vi "PH_Cam_BaseClass.set i Attr and open Services.vi"(0 "i ref in":refnum<vi>, 5 "error in (no error)":errorcluster) -> (14 "i ref out":refnum<vi>, 15 "Image Type":T1 {"Image Type" items=["Grayscale (U8)", "Grayscale (I16)", "Grayscale (SGL)", "Complex (CSG)", "RGB (U32)", "HSL (U32)", "RGB (U64)", "Grayscale (U16)"]}, 16 "i Attributes":T3={"Gui Refs"={"Frame Rate"=refnum, "Get Frame Rate"=refnum, "Show Image"=refnum, "Get Histogram"=refnum, "Mapping"=refnum, "Histogram"=refnum, "Center Cross"=refnum, "Center of Gravity"=refnum, "Scale Factor [%]"=refnum, "Save Image"=refnum, "Palette"=refnum, "Subtract Background"=refnum, "Cam Error"=refnum, "On"=refnum, "Cam List"=refnum}, "Cam"={"Source Notifier"=refnum, "Error"={"status"=FALSE, "code"=0, "source"=""}, "Camera ID"="N/A"}, "Images"={"Cam"=refnum, "Operation"=refnum, "PSDB"=refnum}, "Window Image"={"Indicate Image"=FALSE, "Window No."=0, "Scale Facor"=0.5, "Center Cross"=FALSE, "Subtract Backgr"=FALSE, "CoG"=FALSE, "Color Palette"=[], "Image On"=FALSE}, "Default Prdc Int"=50, "Performance"={"on"=FALSE, "Timestamp Last Frame"=0}, "Histogram"={"on"=FALSE, "Mapping"=FALSE}, "Save Image"={"Save"=FALSE, "File refnum"=refnum}, "Setting Service ID"=0, "Screen"={"x-resolution"=0, "y-resolution"=0}, "On"=FALSE, "Constructor finished"=FALSE, "configured"=FALSE} {"Cam"."Error"."code" format="%.0x"}, 19 "error out":errorcluster)   [LabVIEW 2014, in "PH_Cam_BaseClass.lvlib"]
doc: "In this VI several attributes of this instance are set."
uses:
  PH_Cam_BaseClass.lvlib
  PH_Cam_BaseClass.i attribute.ctl
  PH_Cam_BaseClass.GUI Refs.ctl
  <vilib>/vision/Image Controls.llb/IMAQ Image.ctl
  PH_Cam_BaseClass.Image Type.ctl
  PH_Cam_BaseClass.Settings.ctl
  CSCore/CSSystem/CSSystemLib/CSSystemLib.lvlib
  PH_Common/PH_Common.lvlib
  CSCore/BaseProcess/BaseProcess.lvlib
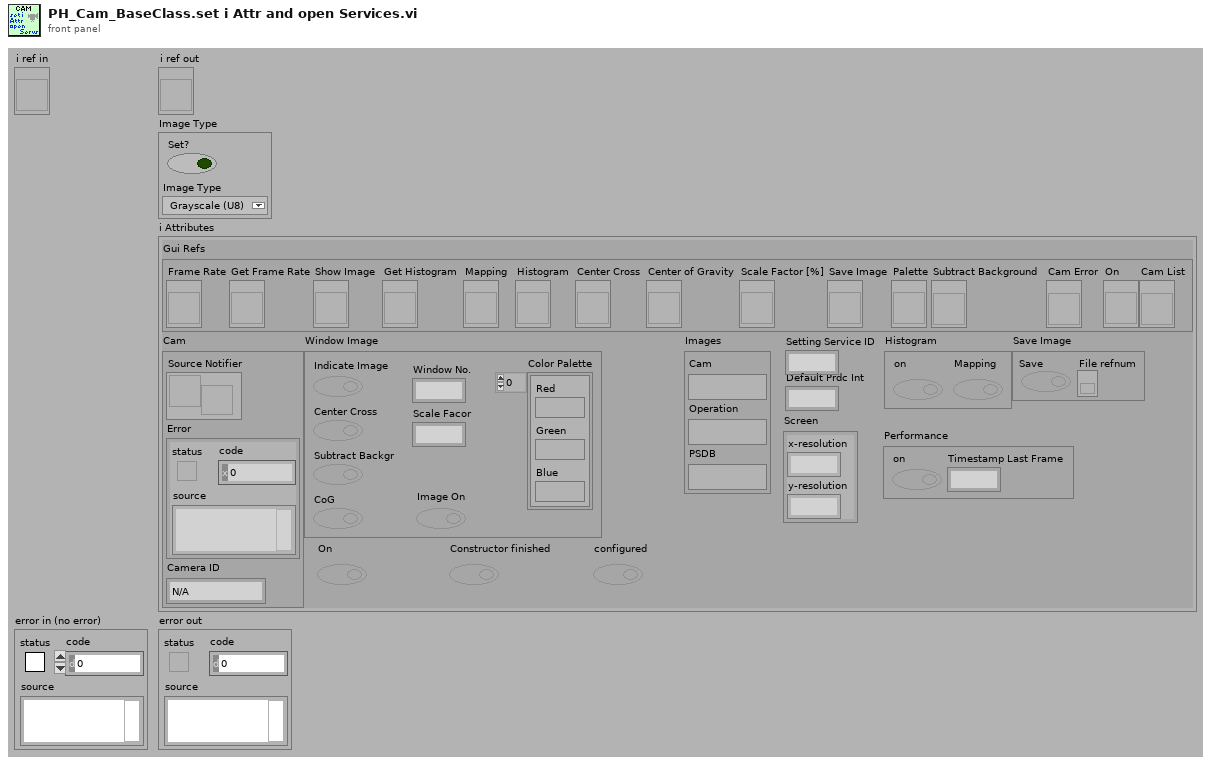
[diagram p1: front panel]
types:
  T1 = typedef "PH_Cam_BaseClass.lvlib/PH_Cam_BaseClass.Image Type.ctl" = cluster{"Set?":bool, "Image Type":T2}
  T2 = typedef "Image Type" = u32
  T3 = typedef "PH_Cam_BaseClass.lvlib/PH_Cam_BaseClass.i attribute.ctl" = cluster{"Gui Refs":T4, "Cam":cluster{"Source Notifier":refnum<notifier>, "Error":errorcluster, "Camera ID":string}, "Images":cluster{"Cam":T5, "Operation":T5, "PSDB":T5}, "Window Image":cluster{"Indicate Image":bool, "Window No.":i32, "Scale Facor":dbl, "Center Cross":bool, "Subtract Backgr":bool, "CoG":bool, "Color Palette":cluster{"Red":u8, "Green":u8, "Blue":u8}[], "Image On":bool}, "Default Prdc Int":i32, "Performance":cluster{"on":bool, "Timestamp Last Frame":i32}, "Histogram":cluster{"on":bool, "Mapping":bool}, "Save Image":cluster{"Save":bool, "File refnum":refnum<file>}, "Setting Service ID":i32, "Screen":cluster{"x-resolution":i16, "y-resolution":i16}, "On":bool, "Constructor finished":bool, "configured":bool}
  T4 = typedef "PH_Cam_BaseClass.lvlib/PH_Cam_BaseClass.GUI Refs.ctl" = cluster{"Frame Rate":refnum<vi>, "Get Frame Rate":refnum<vi>, "Show Image":refnum<vi>, "Get Histogram":refnum<vi>, "Mapping":refnum<vi>, "Histogram":refnum<vi>, "Center Cross":refnum<vi>, "Center of Gravity":refnum<vi>, "Scale Factor [%]":refnum<vi>, "Save Image":refnum<vi>, "Palette":refnum<vi>, "Subtract Background":refnum<vi>, "Cam Error":refnum<vi>, "On":refnum<vi>, "Cam List":refnum<vi>}
  T5 = typedef "IMAQ Image.ctl" = refnum<image>
  T6 = typedef "PH_Cam_BaseClass.lvlib/PH_Cam_BaseClass.Settings.ctl" = cluster{"Cam ID":string, "Gain":dbl, "Brightness":dbl, "Shutter":dbl, "Mode":i32}
  T7 = typedef "LVRectTypeDef.ctl" = cluster{"Left":i16, "Top":i16, "Right":i16, "Bottom":i16}
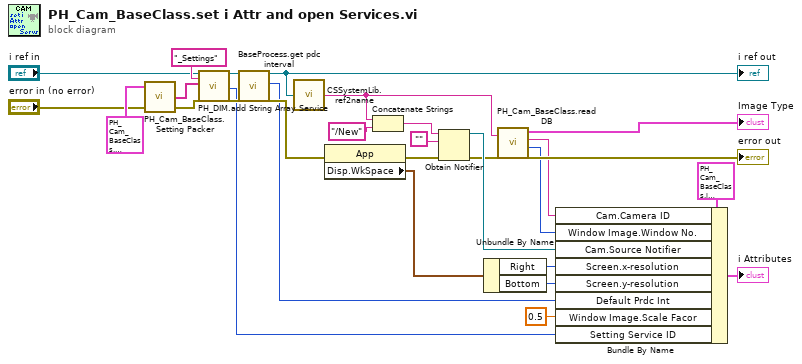
[diagram p0: block diagram]
diagram:
  n1 = call "PH_Cam_BaseClass.Setting Packer.vi"("error in (no error)"="error in (no error)", "Cam Settings In"=T6 {"Cam ID"="123456789123456789", "Gain"=1.2345678912345678e+17, "Brightness"=1.2345678912345678e+17, "Shutter"=1.2345678912345678e+17, "Mode"=2147483647}) -> ("error out"=w15:errorcluster, "Cam Settings"=w16:string[])  [unwired: 1 in, 1 out]
  n2 = call "PH_DIM.add String Array Service.vi"("i ref in"="i ref in", "Service Name"="_Settings", "String Array"=w16, "error in (no error)"=w15) -> ("i ref out"=w12:refnum<vi>, "Service ID"=w8:i32, "error out"=w10:errorcluster)  [unwired: 13 in]
  n3 = call "BaseProcess.get pdc interval.vi"("i ref in"=w12, "error in (no error)"=w10) -> ("i ref out"=w19:refnum<vi>, "PeriodicInterval"=w7:i32, "error out"=w21:errorcluster)  [unwired: 15 in]
  "i ref out" <- w19
  n4 = call "CSSystemLib.ref2name.vi"("obj refnum"=w19) -> ("name"=w6:string)
  n5 = property class="App"(error in=w21) -> (error out=w22:errorcluster, "Disp.WkSpace"=w25:T7)  [unwired: 1 in, 1 out]
  n6 = Concatenate Strings(w6, "/New" ("name (unnamed)")) -> (w29:string)
  n7 = Obtain Notifier(name (unnamed)=w29, notification data type="", error in (no error)=w22) -> (notifier out=w18:refnum<notifier>, error out=w4:errorcluster)  [unwired: 1 in, 1 out]
  n8 = Unbundle By Name(w25) -> ("Right"=w23:i16, "Bottom"=w24:i16)
  n9 = call "PH_Cam_BaseClass.read DB.vi"("DB Entry to read"=w6, "error in (no error)"=w4) -> ("Image Type"=→"Image Type":T1, "Camera ID"=w3:string, "Window Number"=w2:i32, "error out"=→"error out":errorcluster)
  n10 = Bundle By Name(cluster=T3 {"Gui Refs"={"Frame Rate"=refnum, "Get Frame Rate"=refnum, "Show Image"=refnum, "Get Histogram"=refnum, "Mapping"=refnum, "Histogram"=refnum, "Center Cross"=refnum, "Center of Gravity"=refnum, "Scale Factor [%]"=refnum, "Save Image"=refnum, "Palette"=refnum, "Subtract Background"=refnum, "Cam Error"=refnum, "On"=refnum, "Cam List"=refnum}, "Cam"={"Source Notifier"=refnum, "Error"={"status"=FALSE, "code"=0, "source"=""}, "Camera ID"="N/A"}, "Images"={"Cam"=refnum, "Operation"=refnum, "PSDB"=refnum}, "Window Image"={"Indicate Image"=FALSE, "Window No."=0, "Scale Facor"=0.5, "Center Cross"=FALSE, "Subtract Backgr"=FALSE, "CoG"=FALSE, "Color Palette"=[], "Image On"=FALSE}, "Default Prdc Int"=50, "Performance"={"on"=FALSE, "Timestamp Last Frame"=0}, "Histogram"={"on"=FALSE, "Mapping"=FALSE}, "Save Image"={"Save"=FALSE, "File refnum"=refnum}, "Setting Service ID"=0, "Screen"={"x-resolution"=0, "y-resolution"=0}, "On"=FALSE, "Constructor finished"=FALSE, "configured"=FALSE} ("i attribute"), "Cam.Camera ID"=w3, "Window Image.Window No."=w2, "Cam.Source Notifier"=w18, "Screen.x-resolution"=w23, "Screen.y-resolution"=w24, "Default Prdc Int"=w7, "Window Image.Scale Facor"=0.5, "Setting Service ID"=w8) -> (→"i Attributes":T3)
